vi "Start Windows Screen Saver.vi"(8 "error in (no error)":errorcluster) -> (0 "error out":errorcluster)   [LabVIEW 2020, in "MacroAssert.lvlib" / "Winevent.lvlib"]
doc: "This VI will start the Windows screen saver (if installed)."
uses:
  Winevent.lvlib
  Win Util New/Win Util New.lvlib
  user32.dll
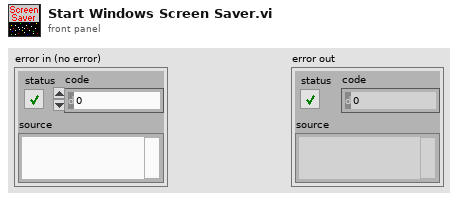
[diagram p1: front panel]
types:
  T1 = enum8{"Maximize Window", "Minimize Window", "Show Task List", "Start Screen Saver", "Quit Application"}
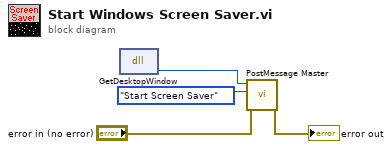
[diagram p0: block diagram]
diagram:
  n1 = dll-call lib="user32.dll" fn="GetDesktopWindow"() -> ("hWndDesktop"=w1:u64)  [unwired: 3 in, 2 out]
  n2 = call "PostMessage Master.vi"("error in"="error in (no error)", "Function"=T1."Start Screen Saver", "window refnum"=w1) -> ("error out"=→"error out":errorcluster)  [unwired: 7 in, 1 out]
